vi "Control Panel.vi"(8 "error in (no error)":errorcluster, 11 "TC in":refnum<class "Temperature Controller.lvclass">) -> (0 "error out":errorcluster, 3 "TC out":refnum<class "Temperature Controller.lvclass">)   [LabVIEW 2012, in "Temperature Controller.lvclass"]
uses:
  Temperature Controller.lvclass
  AutoCtl.ctl
  HV Slide Indicator.ctl
  Utility Classes/InstrPtr/InstrPtr.lvclass
  Temperature Controller.lvclass/Temperature Controller.ctl
  Global/Relative Sound Files.vi
  File IO/File IO.lvclass
  Utility Classes/Readable/Readable.lvclass
panel:
  in  "Timer may start":bool
  in  "Fill VTI":bool
  out "log counter":dbl
  in  "Auto":T1
  in  "SET":bool
  in  "New Temp":dbl[unit]=1.3 min=1.3 max=300.0
  in  "Update interval":dbl[unit]=0.5 min=0.1 max=10.0
  out "*itc503":T2
  out "Currently":dbl[unit]
  in  "Stable Sensitivity +-":dbl=0.05 caption="+/-" min=0.0 step=0.1
  out "stable":bool caption="Stable"
  out "Current Set Point":dbl[unit]=6.0 min=0.0 max=305.0
  out "Internal refresh event signal":bool
  in  "Warn At":dbl[unit]
  in  "Comparison":bool
  in  "Alarm?":bool caption="Boolean"
  in  "Time to Fill":dbl[unit]
  out "Time Remaining":string caption="Time"
  in  "Timer?":bool
  out "done?":bool
  in  "clear":bool
  out "Timer start time":timestamp
  in  "Display":dbl[unit]=600.0
  in  "autoscale?":bool=TRUE
  out "Temperature graph":T3(graph)
  out "active":bool
  out "Auto Indicator":T1={"Auto Heater"=FALSE, "Auto Needle"=FALSE, "Auto PID"=TRUE}
  in  "Auto Controls":T4={"Heater"=FALSE, "Needle"=FALSE, "PID"=TRUE}
  out "Ndisbar":T5 caption="Needle Valve              (est. %)" max=100.0 scale=0.0..100.0 scale format="%.1f"
  in  "Ncontrol":dbl(slide) min=0.0 max=100.0 scale=0.0..100.0
  in  "Hcontrol":dbl(slide) min=0.0 max=99.9 scale=0.0..100.0
  out "Hdispbar":T5 caption="Heater" max=100.0 scale=0.0..100.0 scale format="%.1f"
  out "ready?":bool
  in  "endprgm":bool
  # "Temperature Controller"
  # "This will also open the needle valve,\nif that hasn't already been done."
  # "Greater"
  # "Less"
  # "Manual"
  # "Auto"
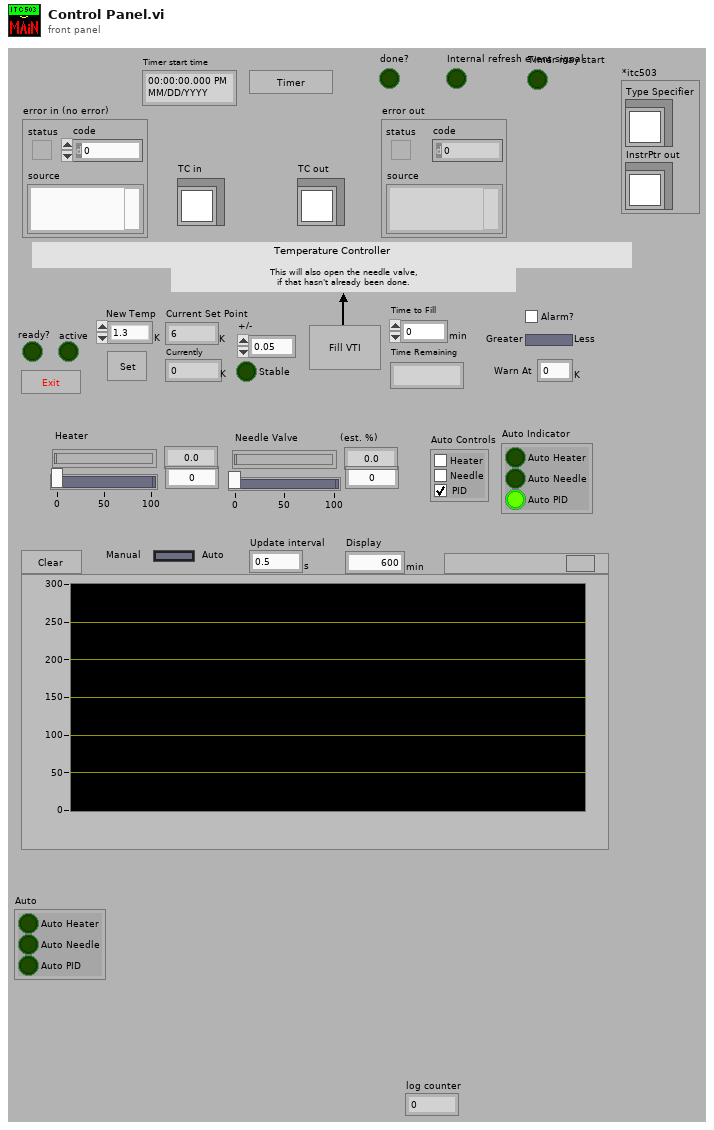
[diagram p1: front panel]
types:
  T1 = typedef "Temperature Controller.lvclass/AutoCtl.ctl" = cluster{"Auto Heater":bool, "Auto Needle":bool, "Auto PID":bool}
  T2 = cluster{"Type Specifier":refnum<class "Temperature Controller.lvclass">, "InstrPtr out":refnum<class "InstrPtr.lvclass">}
  T3 = cluster{"Data Points":cluster{"t":timestamp, "x":dbl}[]}[]
  T4 = cluster{"Heater":bool, "Needle":bool, "PID":bool}
  T5 = typedef "Temperature Controller.lvclass/HV Slide Indicator.ctl" = dbl
  T6 = enum8{"Enabled", "Disabled", "Disabled and Grayed Out"}
  T7 = cluster{"Temperature Controller out":refnum<class "Temperature Controller.lvclass">, "Instrument Pointer":refnum<class "InstrPtr.lvclass">}
  T8 = typedef "ITCIO.ctl" = cluster{"Address":T9, "Version":T10, "Ch 1 dec places":i16, "Ch 2 dec places":i16, "Ch 3 dec places":i16, "Ch1 Name":string, "Ch2 Name":string, "Ch3 Name":string}
  T9 = typedef "OxfordAddress.ctl" = cluster{"Com Port":i32, "ISOBUS Address":i32, "GPIB Address":i16, "Communication":enum16{"RS232", "ISOBUS", "GPIB", "Gateway"}}
  T10 = typedef "ITCVersion.ctl" = enum16{"ITC502", "ITC503", "ITC601"}
  T11 = typedef "Readable.lvclass/TX Graph.ctl" = cluster{"Data Points":cluster{"t":timestamp, "x":dbl}[]}[]
  T12 = cluster{"Data Points":cluster{"t":timestamp, "x":dbl}[]}
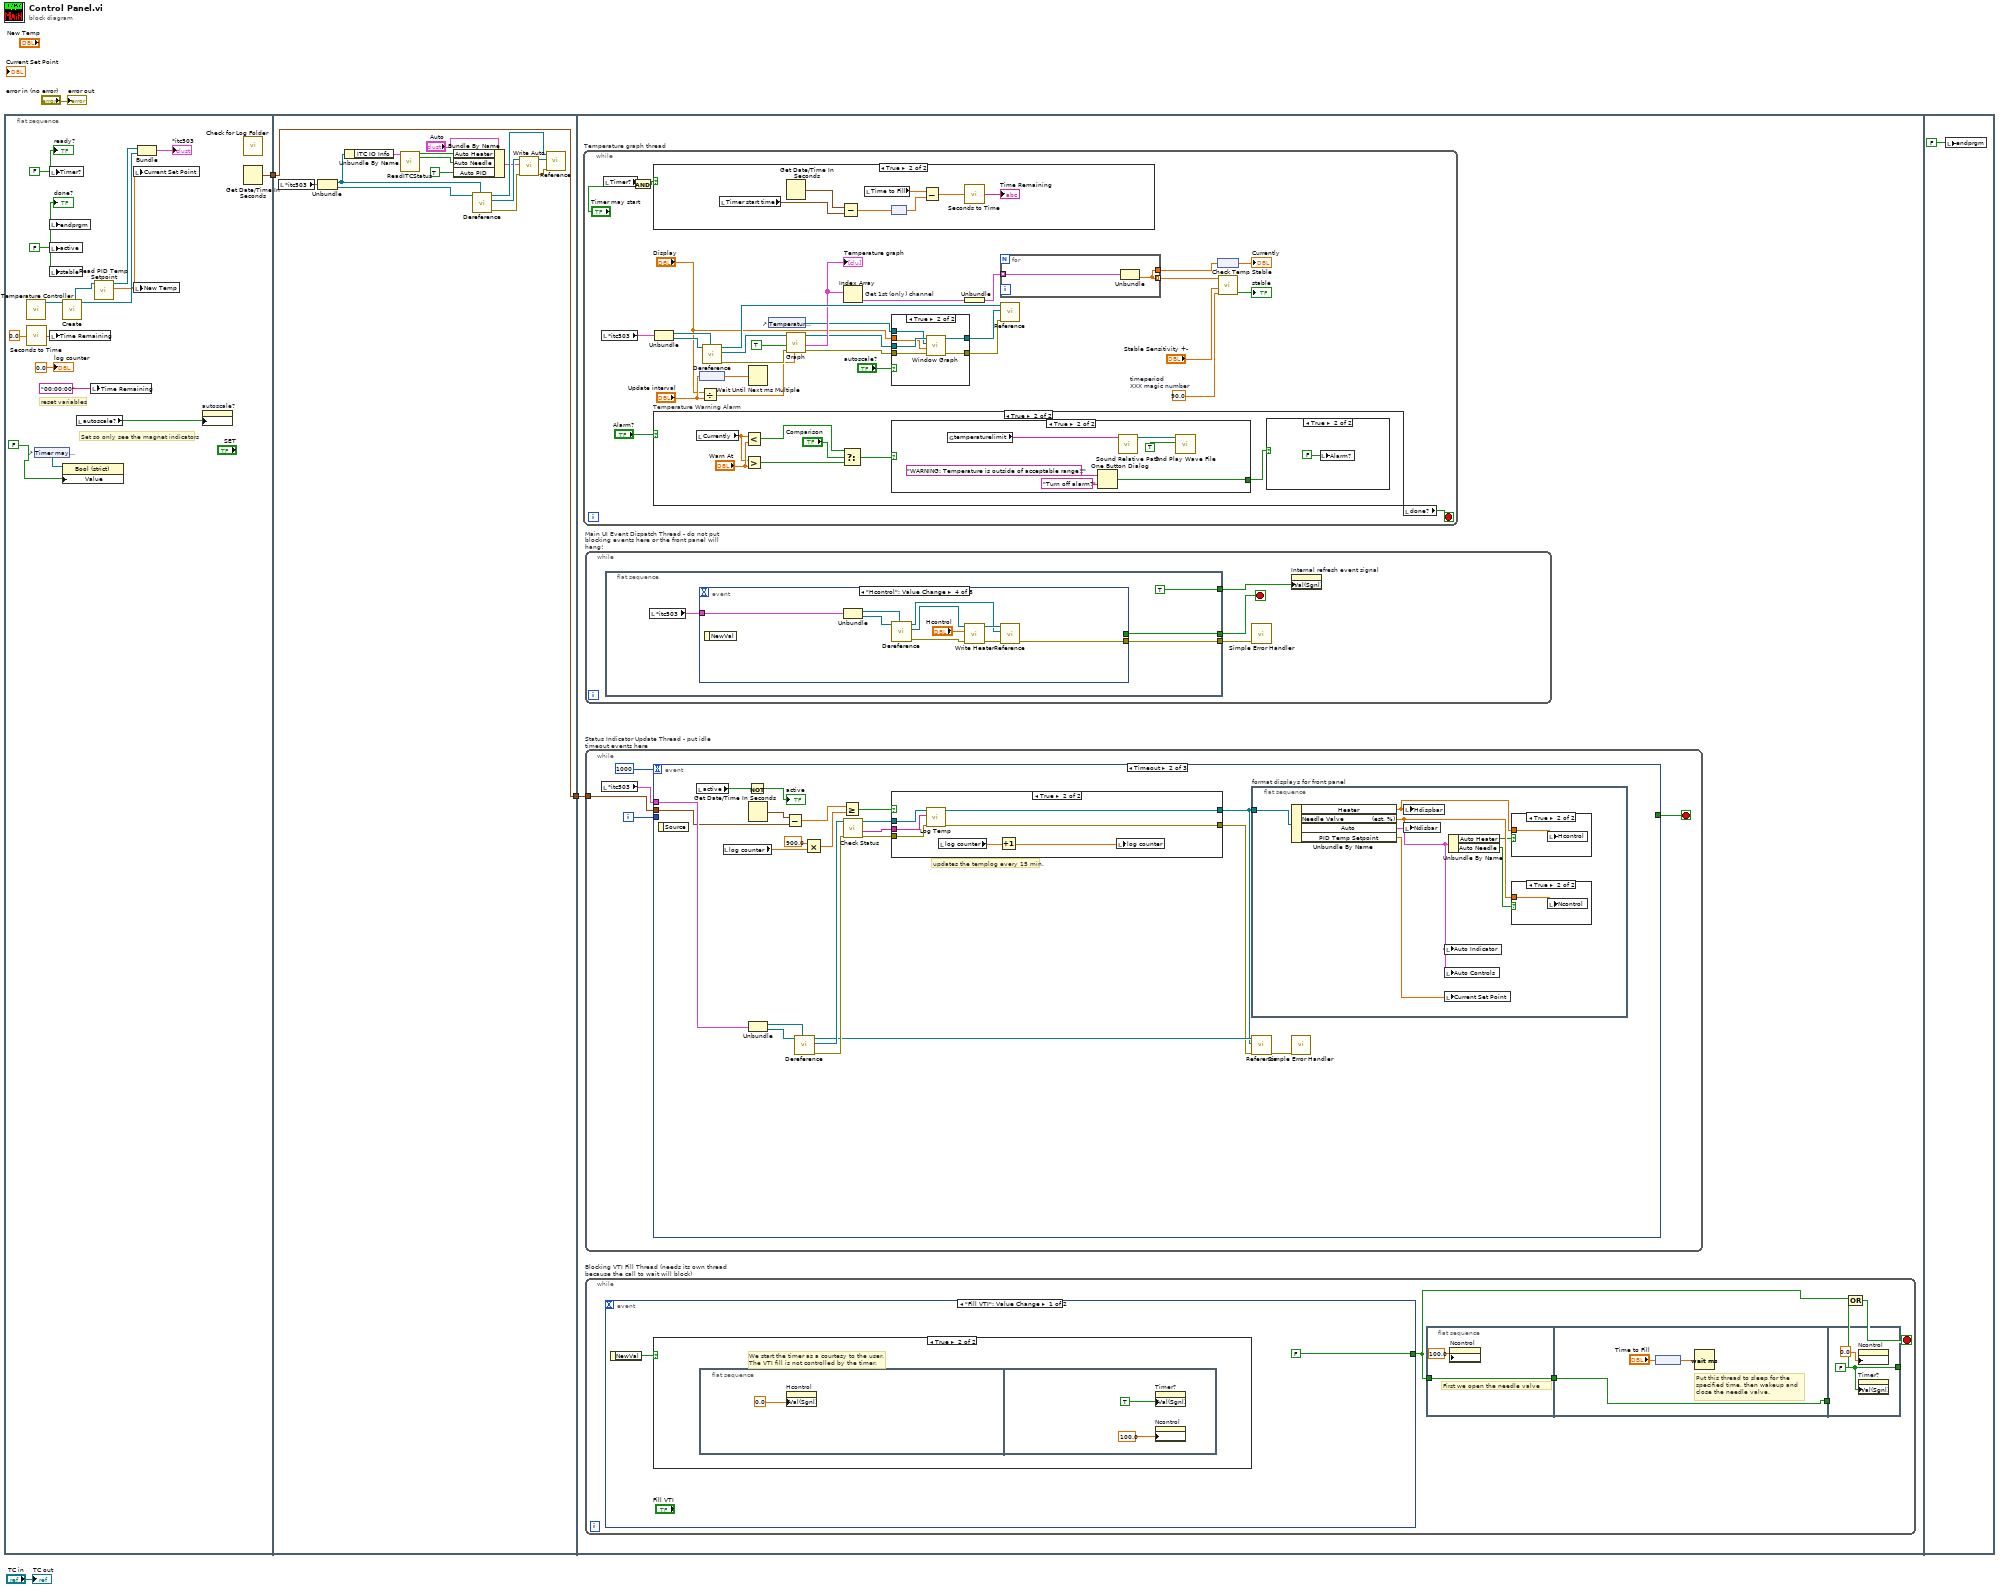
[diagram p0: block diagram]
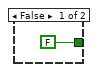
[diagram p6: hidden frame]
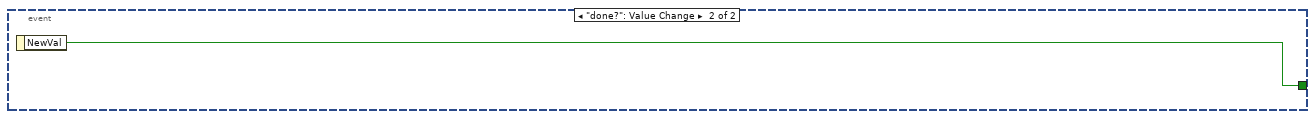
[diagram p8: hidden frame]
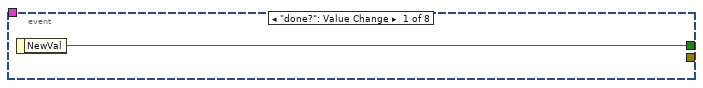
[diagram p9: hidden frame]
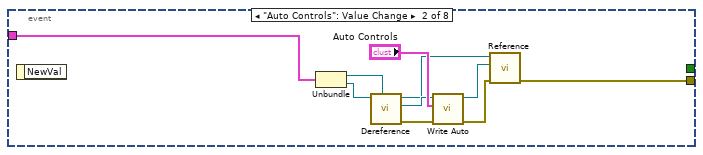
[diagram p10: hidden frame]
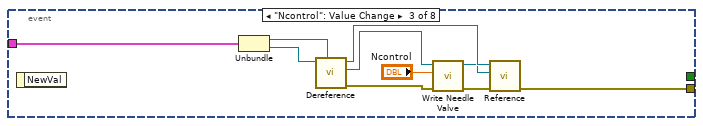
[diagram p11: hidden frame]
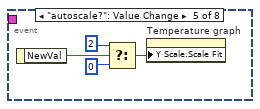
[diagram p12: hidden frame]
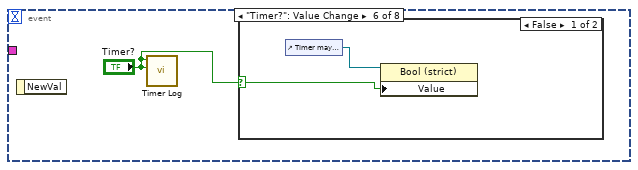
[diagram p13: hidden frame]
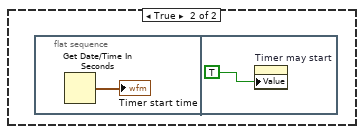
[diagram p14: hidden frame]
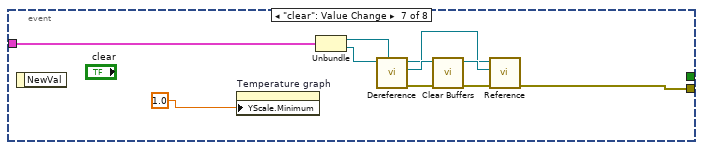
[diagram p15: hidden frame]
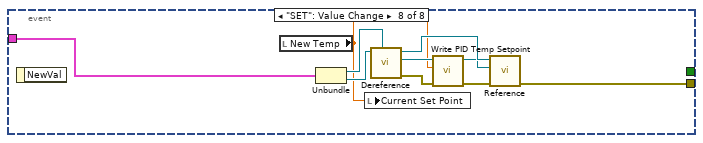
[diagram p16: hidden frame]
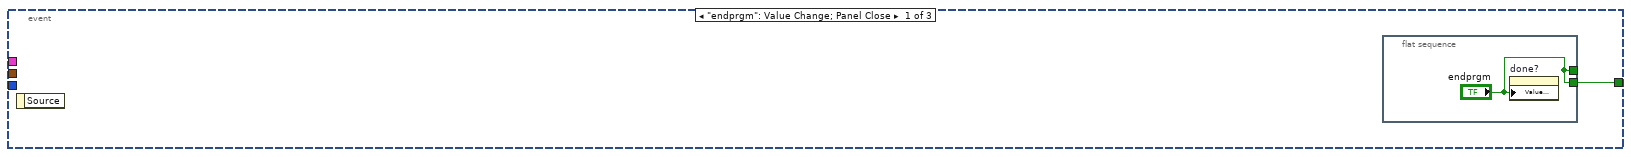
[diagram p17: hidden frame]
diagram:
  n1 = flat-sequence {
    tunnel: [w9] -> w2
    tunnel: w2 -> [w21]
    tunnel: [w21] -> w1
    tunnel: w1 -> [w36]
    frame #0 {
      w20 = FALSE
      w17 = FALSE
      # "Set so only see the magnet indicators"
      # "reset variables"
      n2 = call "Temperature Controller.vi"() -> ("Temperature Controller out"=w16:refnum<class "Temperature Controller.lvclass">)  [unwired: 10 in, 1 out]
      n3 = call "Seconds to Time.vi"("Seconds"=dbl[unit] 0.0) -> ("Time"=w13:string)
      n4 = control-ref of="Timer may start"() -> (w5:refnum<vi>)
      n5 = local write "Timer?"(w20) -> ()
      n6 = local write "endprgm"(w17) -> ()
      n7 = local write "active"(w17) -> ()
      n8 = local write "stable"(w17) -> ()
      n9 = local write "Time Remaining"(w13) -> ()
      n10 = call "Create.vi"("Instrument in"=w16) -> ("Instrument Pointer"=w15:refnum<class "InstrPtr.lvclass">, "Type Specifier"=w11:refnum<class "Temperature Controller.lvclass">)  [unwired: 8 in, 1 out]
      n11 = property on="Property Node" class="Bool (strict)"(reference=w5, "Value"=FALSE) -> ()  [unwired: 1 in, 2 out]
      n12 = local read "autoscale?"() -> (w18:bool)
      n13 = local write "Time Remaining"("00:00:00") -> ()
      n14 = call-dynamic "Read PID Temp Setpoint.vi"("Temperature Controller in"=w11) -> ("PID Temp Setpoint"=w7:dbl[unit], "Temperature Controller out"=w10:refnum<class "Temperature Controller.lvclass">)  [unwired: 8 in, 1 out]
      n15 = local write "Current Set Point"(w7) -> ()
      n16 = local write "New Temp"(w7) -> ()
      n17 = Bundle("Temperature Controller out"=w10, "Instrument Pointer"=w15) -> (→"*itc503":T7)  [unwired: 1 in]
      n18 = property on="autoscale?" class="Bool (strict)"("Value (Signaling)"=w18) -> ()  [unwired: 2 in, 2 out]
      n19 = call "Check for Log Folder.vi"() -> ()  [unwired: 1 out]
      n20 = Get Date/Time In Seconds() -> (seconds since 1Jan1904=w9:timestamp)
      "ready?" <- w20
      "done?" <- w17
      "log counter" <- 0.0 ("log counter")
    }
    frame #1 {
      n21 = local read "*itc503"() -> (w35:T2)
      n22 = Unbundle(w35) -> ("Type Specifier"=w24:refnum<class "Temperature Controller.lvclass">, "InstrPtr out"=w29:refnum<class "InstrPtr.lvclass">)
      n23 = Unbundle By Name(w24) -> ("ITC IO Info"=w23:T8)
      n24 = call "ReadITCStatus.vi"("ITC IO Info"=w23) -> ("Auto heat"=w26:bool, "Auto Needle Valve"=w25:bool)  [unwired: 13 out]
      n25 = Bundle By Name(cluster="Auto", "Auto Heater"=w26, "Auto Needle"=w25, "Auto PID"=TRUE) -> (w27:T1)
      n26 = call "Dereference.vi"("Type Specifier"=w24, "InstrPtr"=w29) -> ("error out"=w34:errorcluster, "Instrument out"=w32:refnum<class "Temperature Controller.lvclass">, "InstrPtr out"=w31:refnum<class "InstrPtr.lvclass">)  [unwired: 7 in]
      n27 = call-dynamic "Write Auto.vi"("error in (no error)"=w34, "Auto"=w27, "Temperature Controller in"=w32) -> ("error out"=w33:errorcluster, "Temperature Controller out"=w30:refnum<class "Temperature Controller.lvclass">)  [unwired: 7 in]
      n28 = call "Reference.vi"("error in (no error)"=w33, "Instrument"=w30, "InstrPtr in"=w31) -> ()  [unwired: 8 in, 1 out]
    }
    frame #2 {
      n29 = while "Temperature graph thread" {
        stop <- w48 stop-if-true
        w60 = 90.0  # timeperiod XXX magic number
        n30 = local read "*itc503"() -> (w56:T2)
        n31 = local read "Timer?"() -> (w49:bool)
        n32 = And(x=w49, y="Timer may start") -> (x .and. y?=w38:bool)
        n33 = case shown="True" w38 {
          frame False {
          }
          frame True {
            n34 = local read "Timer start time"() -> (w73:timestamp)
            n35 = Get Date/Time In Seconds ("jkl;jkljkl")() -> (seconds since 1Jan1904=w74:timestamp)
            n36 = Subtract(x=w74, y=w73) -> (x-y=w76:dbl)
            n37 = local read "Time to Fill"() -> (w70:dbl[unit])
            n38 = node(w76) -> (w72:dbl[unit])
            n39 = Subtract(x=w70, y=w72) -> (x-y=w71:dbl[unit])
            n40 = call "Seconds to Time.vi"("Seconds"=w71) -> ("Time"=→"Time Remaining":string)
          }
        }
        n41 = case "Temperature Warning Alarm" shown="True" "Alarm?" {
          frame False {
          }
          frame True {
            n42 = local read "Currently"() -> (w86:dbl[unit])
            n43 = Less?(x=w86, y="Warn At") -> (x < y?=w90:bool)
            n44 = Greater?(x=w86, y="Warn At") -> (0:w89:bool)
            n45 = Select(t=w90, s="Comparison", f=w89) -> (s? t:f=w88:bool)
            n46 = case shown="True" w88 {
              tunnel: [FALSE ("true") w95] -> w85
              frame False {
              }
              frame True {
                n47 = global read "Relative Sound Files.vi" "temperaturelimit"() -> (w98:string)
                n48 = One Button Dialog(message="WARNING: Temperature is outside of acceptable range!!", button name ("OK")="Turn off alarm?") -> (true=w95:bool)
                n49 = call "Sound Relative Path.vi"("Sound"=w98) -> ("Relative Path"=w97:path)  [unwired: 10 in]
                n50 = call <vilib>:"Snd Play Wave File.vi"("wait until finish (T)"=TRUE, "wave file path"=w97) -> ()  [unwired: 1 in, 9 out]
              }
            }
            n51 = case shown="True" w85 {
              frame False {
              }
              frame True {
                n52 = local write "Alarm?"(FALSE ("Alarm?")) -> ()
              }
            }
          }
        }
        n53 = Unbundle(w56) -> ("Type Specifier"=w61:refnum<class "Temperature Controller.lvclass">, "InstrPtr out"=w62:refnum<class "InstrPtr.lvclass">)
        n54 = node("Update interval") -> (w47:dbl)
        n55 = Divide(x="Display", y="Update interval") -> (x/y=w45:dbl)
        n56 = call "Dereference.vi"("Type Specifier"=w61, "InstrPtr"=w62) -> ("error out"=w65:errorcluster, "Instrument out"=w64:refnum<class "Temperature Controller.lvclass">, "InstrPtr out"=w63:refnum<class "InstrPtr.lvclass">)  [unwired: 7 in]
        n57 = Wait Until Next ms Multiple(millisecond multiple=w47) -> ()  [unwired: 1 out]
        n58 = control-ref of="Temperature graph"() -> (w40:refnum<vi>)
        n59 = call-dynamic "Graph.vi"("Ring size (points) (1024)"=w45, "error in (no error)"=w65, "Store Ring? (f)"=TRUE, "Readable in"=w64) -> ("error out"=w44:errorcluster, "Ring Buffers"=w55:T11, "Readable out"=w43:refnum<class "Temperature Controller.lvclass">)  [unwired: 1 in, 4 out]
        "Temperature graph" <- w55
        n60 = Index Array "Get 1st (only) channel"(array=w55) -> (element=w54:T12)  [unwired: 1 in]
        n61 = case shown="True" "autoscale?" {
          tunnel: w44 -> [w77 w84]
          tunnel: w43 -> [w78 w83]
          tunnel: [w78 w82] -> w42
          tunnel: [w77 w81] -> w41
          tunnel: w40 -> [_ w80]
          tunnel: "Display" -> [_ w79]
          frame False {
          }
          frame True {
            n62 = call-dynamic "Window Graph.vi"("error in (no error)"=w84, "Window"=w79, "Graph ref"=w80, "Readable in"=w83) -> ("error out"=w81:errorcluster, "Readable out"=w82:refnum<class "Temperature Controller.lvclass">)  [unwired: 6 in]
          }
        }
        n63 = Unbundle(w54) -> ("Data Points"=w53:cluster{"t":timestamp, "x":dbl}[])
        n64 = for {
          tunnel: w53 -> [w69] mode=indexing
          tunnel: [w68] -> w52 mode=indexing
          tunnel: [w68] -> w51
          n65 = Unbundle(w69) -> ("x"=w68:dbl)  [unwired: 1 out]
        }
        n66 = call "Reference.vi"("error in (no error)"=w41, "Instrument"=w42, "InstrPtr in"=w63) -> ()  [unwired: 8 in, 1 out]
        n67 = node(w51) -> (→"Currently":dbl[unit])
        n68 = call "Check Temp Stable.vi"("timeperiod"=w60, "sens"="Stable Sensitivity +-", "temparray"=w52) -> ("stable"=→"stable":bool)  [unwired: 8 in]
        n69 = local read "done?"() -> (w48:bool)
      }
      n70 = while "Main UI Event Dispatch Thread - do not put blocking events here or the front panel will hang!" {
        stop <- w120 stop-if-true
        n71 = flat-sequence {
          tunnel: [w124] -> w119
          tunnel: [w123] -> w120
          tunnel: [TRUE ("Value (Signaling)")] -> w118
          frame #0 {
            n72 = local read "*itc503"() -> (w122:T2)
            n73 = event shown="[3] \"Hcontrol\": Value Change" {
              selector: _ -> [_ _ _ _ _ _ _ _]
              dyn-events: _ -> [_ _ _ _ _ _ _ _]
              timeout: _ -> [_ _ _ _ _ _ _ _]
              tunnel: [w125 _ _ _ _ _ _ _] -> w123
              tunnel: w122 -> [_ w131 w142 w151 _ _ w169 w181]
              tunnel: [_ w132 w143 w152 _ _ w166 w182] -> w124
              event "done?": Value Change {
                n74 = event-data() -> ("NewVal"=w125:bool)  [unwired: 1 out]
              }
              event "Auto Controls": Value Change {
                n75 = event-data() -> ()  [unwired: 2 out]
                n76 = Unbundle(w131) -> ("Type Specifier"=w127:refnum<class "Temperature Controller.lvclass">, "InstrPtr out"=w126:refnum<class "InstrPtr.lvclass">)
                n77 = call "Dereference.vi"("Type Specifier"=w127, "InstrPtr"=w126) -> ("error out"=w134:errorcluster, "Instrument out"=w130:refnum<class "Temperature Controller.lvclass">, "InstrPtr out"=w129:refnum<class "InstrPtr.lvclass">)  [unwired: 7 in]
                n78 = call-dynamic "Write Auto.vi"("error in (no error)"=w134, "Auto"="Auto Controls", "Temperature Controller in"=w130) -> ("error out"=w133:errorcluster, "Temperature Controller out"=w128:refnum<class "Temperature Controller.lvclass">)  [unwired: 7 in]
                n79 = call "Reference.vi"("error in (no error)"=w133, "Instrument"=w128, "InstrPtr in"=w129) -> ("error out"=w132:errorcluster)  [unwired: 8 in]
              }
              event "Ncontrol": Value Change {
                n80 = event-data() -> ()  [unwired: 2 out]
                n81 = Unbundle(w142) -> ("Type Specifier"=w138:refnum<class "Temperature Controller.lvclass">, "InstrPtr out"=w137:refnum<class "InstrPtr.lvclass">)
                n82 = call "Dereference.vi"("Type Specifier"=w138, "InstrPtr"=w137) -> ("error out"=w144:errorcluster, "Instrument out"=w141:refnum<class "Temperature Controller.lvclass">, "InstrPtr out"=w140:refnum<class "InstrPtr.lvclass">)  [unwired: 7 in]
                n83 = call-dynamic "Write Needle Valve.vi"("error in (no error)"=w144, "Heater"="Ncontrol", "Temperature Controller in"=w141) -> ("error out"=w145:errorcluster, "Temperature Controller out"=w139:refnum<class "Temperature Controller.lvclass">)  [unwired: 7 in]
                n84 = call "Reference.vi"("error in (no error)"=w145, "Instrument"=w139, "InstrPtr in"=w140) -> ("error out"=w143:errorcluster)  [unwired: 8 in]
              }
              event "Hcontrol": Value Change {
                n85 = event-data() -> ()  [unwired: 2 out]
                n86 = Unbundle(w151) -> ("Type Specifier"=w146:refnum<class "Temperature Controller.lvclass">, "InstrPtr out"=w147:refnum<class "InstrPtr.lvclass">)
                n87 = call "Dereference.vi"("Type Specifier"=w146, "InstrPtr"=w147) -> ("error out"=w154:errorcluster, "Instrument out"=w150:refnum<class "Temperature Controller.lvclass">, "InstrPtr out"=w149:refnum<class "InstrPtr.lvclass">)  [unwired: 7 in]
                n88 = call-dynamic "Write Heater.vi"("error in (no error)"=w154, "Heater"="Hcontrol", "Temperature Controller in"=w150) -> ("error out"=w153:errorcluster, "Temperature Controller out"=w148:refnum<class "Temperature Controller.lvclass">)  [unwired: 7 in]
                n89 = call "Reference.vi"("error in (no error)"=w153, "Instrument"=w148, "InstrPtr in"=w149) -> ("error out"=w152:errorcluster)  [unwired: 8 in]
              }
              event "autoscale?": Value Change {
                n90 = event-data() -> ("NewVal"=w156:bool)  [unwired: 1 out]
                n91 = Select(t=2, s=w156, f=0) -> (s? t:f=w159:i32)
                n92 = property on="Temperature graph" class="XYGraph (strict)"("Y Scale.Scale Fit"=w159) -> ()  [unwired: 2 in, 2 out]
              }
              event "Timer?": Value Change {
                n93 = event-data() -> ()  [unwired: 2 out]
                n94 = call "Timer Log.vi"("flag"="Timer?", "toggle"="Timer?") -> ()  [unwired: 10 out]
                n95 = case shown="False" "Timer?" {
                  selector: "Timer?" -> [w162 _]
                  frame False {
                    n96 = control-ref of="Timer may start"() -> (w161:refnum<vi>)
                    n97 = property on="Property Node" class="Bool (strict)"(reference=w161, "Value"=w162) -> ()  [unwired: 1 in, 2 out]
                  }
                  frame True {
                    n98 = flat-sequence {
                      frame #0 {
                        n99 = Get Date/Time In Seconds() -> (seconds since 1Jan1904=→"Timer start time":timestamp)
                      }
                      frame #1 {
                        n100 = property on="Timer may start" class="Bool (strict)"("Value"=TRUE ("Value (Signaling)")) -> ()  [unwired: 2 in, 2 out]
                      }
                    }
                  }
                }
              }
              event "clear": Value Change {
                n101 = event-data() -> ()  [unwired: 2 out]
                n102 = property on="Temperature graph" class="XYGraph (strict)"("YScale.Minimum"=1.0) -> ()  [unwired: 2 in, 2 out]
                n103 = Unbundle(w169) -> ("Type Specifier"=w170:refnum<class "Temperature Controller.lvclass">, "InstrPtr out"=w171:refnum<class "InstrPtr.lvclass">)
                n104 = call "Dereference.vi"("Type Specifier"=w170, "InstrPtr"=w171) -> ("error out"=w168:errorcluster, "Instrument out"=w174:refnum<class "Temperature Controller.lvclass">, "InstrPtr out"=w172:refnum<class "InstrPtr.lvclass">)  [unwired: 7 in]
                n105 = call "Clear Buffers.vi"("error in (no error)"=w168, "Readable in"=w174) -> ("error out"=w167:errorcluster, "Readable out"=w173:refnum<class "Temperature Controller.lvclass">)  [unwired: 8 in]
                n106 = call "Reference.vi"("error in (no error)"=w167, "Instrument"=w173, "InstrPtr in"=w172) -> ("error out"=w166:errorcluster)  [unwired: 8 in]
              }
              event "SET": Value Change {
                n107 = event-data() -> ()  [unwired: 2 out]
                n108 = local read "New Temp"() -> (w175:dbl[unit])
                n109 = Unbundle(w181) -> ("Type Specifier"=w177:refnum<class "Temperature Controller.lvclass">, "InstrPtr out"=w176:refnum<class "InstrPtr.lvclass">)
                n110 = local write "Current Set Point"(w175) -> ()
                n111 = call "Dereference.vi"("Type Specifier"=w177, "InstrPtr"=w176) -> ("error out"=w183:errorcluster, "Instrument out"=w179:refnum<class "Temperature Controller.lvclass">, "InstrPtr out"=w180:refnum<class "InstrPtr.lvclass">)  [unwired: 7 in]
                n112 = call-dynamic "Write PID Temp Setpoint.vi"("error in (no error)"=w183, "PID Temp Setpoint"=w175, "Temperature Controller in"=w179) -> ("error out"=w184:errorcluster, "Temperature Controller out"=w178:refnum<class "Temperature Controller.lvclass">)  [unwired: 7 in]
                n113 = call "Reference.vi"("error in (no error)"=w184, "Instrument"=w178, "InstrPtr in"=w180) -> ("error out"=w182:errorcluster)  [unwired: 8 in]
              }
            }
          }
        }
        n114 = call <vilib>:"Simple Error Handler.vi"("error in (no error)"=w119) -> ()  [unwired: 4 in, 5 out]
        n115 = property on="Internal refresh event signal" class="Bool (strict)"("Val(Sgnl)"=w118) -> ()  [unwired: 2 in, 2 out]
      }
      n116 = while "Status Indicator Update Thread - put idle timeout events here" {
        tunnel: w36 -> [w185]
        i -> [w187]
        stop <- w188 stop-if-true
        n117 = local read "*itc503"() -> (w186:T2)
        n118 = event shown="[1] Timeout" {
          selector: _ -> [_ _ _]
          dyn-events: _ -> [_ _ _]
          timeout: 1000 -> [_ _ _]
          tunnel: [w190 _ _] -> w188
          tunnel: w187 -> [_ _ _]
          tunnel: w186 -> [_ w210 w239]
          tunnel: w185 -> [_ w196 _]
          event "endprgm": Value Change; Panel Close {
            n119 = event-data() -> ()  [unwired: 2 out]
            n120 = flat-sequence {
              tunnel: ["endprgm"] -> _
              tunnel: ["endprgm"] -> w190
              frame #0 {
                n121 = property on="done?" class="Bool (strict)"("Value (Signaling)"="endprgm") -> ()  [unwired: 2 in, 2 out]
              }
            }
          }
          event Timeout {
            # "updates the templog every 15 min."
            n122 = event-data() -> ()  [unwired: 2 out]
            n123 = local read "active"() -> (w212:bool)
            n124 = local read "log counter"() -> (w194:dbl)
            n125 = Not(x=w212) -> (.not. x?=→"active":bool)
            n126 = Get Date/Time In Seconds() -> (seconds since 1Jan1904=w197:timestamp)
            n127 = Unbundle(w210) -> ("Type Specifier"=w206:refnum<class "Temperature Controller.lvclass">, "InstrPtr out"=w207:refnum<class "InstrPtr.lvclass">)
            n128 = Subtract(x=w197, y=w196) -> (x-y=w192:dbl)
            n129 = call "Dereference.vi"("Type Specifier"=w206, "InstrPtr"=w207) -> ("error out"=w209:errorcluster, "Instrument out"=w208:refnum<class "Temperature Controller.lvclass">, "InstrPtr out"=w205:refnum<class "InstrPtr.lvclass">)  [unwired: 7 in]
            n130 = Multiply(x=900.0 ("y"), y=w194) -> (x*y=w193:dbl)
            n131 = Greater Or Equal?(x=w192, y=w193) -> (x >= y?=w199:bool)
            n132 = call-dynamic "Check Status.vi"("error in (no error)"=w209, "Temperature Controller in"=w208) -> ("error out"=w202:errorcluster, "Status"=w198:string, "Temperature Controller out"=w204:refnum<class "Temperature Controller.lvclass">)  [unwired: 6 in, 1 out]
            n133 = case shown="True" w199 {
              tunnel: w204 -> [w214 w221]
              tunnel: [w214 w220] -> w203
              tunnel: w202 -> [w213 w219]
              tunnel: [w213 w218] -> w201
              tunnel: w198 -> [_ w217]
              frame False {
              }
              frame True {
                n134 = call-dynamic "Log Temp.vi"("error in (no error)"=w219, "Status string"=w217, "Temperature Controller in"=w221) -> ("error out"=w218:errorcluster, "Temperature Controller out"=w220:refnum<class "Temperature Controller.lvclass">)  [unwired: 7 in]
                n135 = local read "log counter"() -> (w216:dbl)
                n136 = Increment(x=w216) -> (x+1=w215:dbl)
                n137 = local write "log counter"(w215) -> ()
              }
            }
            n138 = flat-sequence "format displays for front panel" {
              tunnel: w203 -> [w228]
              frame #0 {
                n139 = Unbundle By Name(w228) -> ("Heater"=w226:T5, "Needle Valve              (est. %)"=w225:T5, "Auto"=w224:T1, "PID Temp Setpoint"=w227:dbl[unit])
                n140 = local write "Hdispbar"(w226) -> ()
                n141 = local write "Ndisbar"(w225) -> ()
                n142 = local write "Auto Indicator"(w224) -> ()
                n143 = local write "Auto Controls"(w224) -> ()
                n144 = local write "Current Set Point"(w227) -> ()
                n145 = Unbundle By Name(w224) -> ("Auto Heater"=w223:bool, "Auto Needle"=w222:bool)
                n146 = case shown="True" w223 {
                  tunnel: w226 -> [_ w230]
                  frame False {
                  }
                  frame True {
                    n147 = local write "Hcontrol"(w230) -> ()
                  }
                }
                n148 = case shown="True" w222 {
                  tunnel: w225 -> [_ w229]
                  frame False {
                  }
                  frame True {
                    n149 = local write "Ncontrol"(w229) -> ()
                  }
                }
              }
            }
            n150 = call "Reference.vi"("error in (no error)"=w201, "Instrument"=w203, "InstrPtr in"=w205) -> ("error out"=w200:errorcluster)  [unwired: 8 in]
            n151 = call <vilib>:"Simple Error Handler.vi"("error in (no error)"=w200) -> ()  [unwired: 4 in, 5 out]
          }
          event "Internal refresh event signal": Value Change {
            # "min = max - window\nmax = now"
            # "read indicators"
            # "check whats on and read settings"
            n152 = event-data() -> ()  [unwired: 2 out]
            n153 = Unbundle(w239) -> ("Type Specifier"=w237:refnum<class "Temperature Controller.lvclass">, "InstrPtr out"=w236:refnum<class "InstrPtr.lvclass">)
            n154 = call "Dereference.vi"("Type Specifier"=w237, "InstrPtr"=w236) -> ("error out"=w233:errorcluster, "Instrument out"=w235:refnum<class "Temperature Controller.lvclass">, "InstrPtr out"=w234:refnum<class "InstrPtr.lvclass">)  [unwired: 7 in]
            n155 = call-dynamic "Check Status.vi"("error in (no error)"=w233, "Temperature Controller in"=w235) -> ("error out"=w232:errorcluster, "Ready?"=w238:bool, "Temperature Controller out"=w231:refnum<class "Temperature Controller.lvclass">)  [unwired: 6 in, 1 out]
            n156 = local write "ready?"(w238) -> ()
            n157 = call "Reference.vi"("error in (no error)"=w232, "Instrument"=w231, "InstrPtr in"=w234) -> ()  [unwired: 8 in, 1 out]
            n158 = flat-sequence "format displays for front panel" {
              tunnel: w231 -> [w245]
              frame #0 {
                n159 = Unbundle By Name(w245) -> ("Heater"=w249:T5, "Needle Valve              (est. %)"=w246:T5, "Auto"=w248:T1, "PID Temp Setpoint"=w244:dbl[unit])
                "Auto Indicator" <- w248
                "Ndisbar" <- w246
                "Hdispbar" <- w249
                n160 = local write "Auto Controls"(w248) -> ()
                n161 = local write "Current Set Point"(w244) -> ()
                n162 = Unbundle By Name(w248) -> ("Auto Heater"=w250:bool)
                n163 = Unbundle By Name(w248) -> ("Auto Needle"=w247:bool)
                n164 = case shown="True" w250 {
                  tunnel: w249 -> [_ w252]
                  frame False {
                  }
                  frame True {
                    n165 = local write "Hcontrol"(w252) -> ()
                  }
                }
                n166 = case shown="True" w247 {
                  tunnel: w246 -> [_ w251]
                  frame False {
                  }
                  frame True {
                    n167 = local write "Ncontrol"(w251) -> ()
                  }
                }
              }
            }
            n168 = flat-sequence "Disable controls if unit is powered off" {
              tunnel: w238 -> [w242]
              frame #0 {
                n169 = Select(t=T6."Enabled" ("Disabled"), s=w242, f=T6."Disabled and Grayed Out" ("Disabled")) -> (s? t:f=w243:T6)
                n170 = property on="Current Set Point" class="DigNum (strict)"("Disabled"=w243) -> ()  [unwired: 2 in, 2 out]
                n171 = property on="Hdispbar" class="Slide (strict)"("Disabled"=w243) -> ()  [unwired: 2 in, 2 out]
                n172 = property on="Hcontrol" class="Slide (strict)"("Disabled"=w243) -> ()  [unwired: 2 in, 2 out]
                n173 = property on="Ncontrol" class="Slide (strict)"("Disabled"=w243) -> ()  [unwired: 2 in, 2 out]
                n174 = property on="Ndisbar" class="Slide (strict)"("Disabled"=w243) -> ()  [unwired: 2 in, 2 out]
                n175 = property on="Stable Sensitivity +-" class="DigNum (strict)"("Disabled"=w243) -> ()  [unwired: 2 in, 2 out]
                n176 = property on="Auto Controls" class="Clust (strict)"("Disabled"=w243) -> ()  [unwired: 2 in, 2 out]
                n177 = property on="Auto Indicator" class="Clust (strict)"("Disabled"=w243) -> ()  [unwired: 2 in, 2 out]
                n178 = property on="stable" class="Bool (strict)"("Disabled"=w243) -> ()  [unwired: 2 in, 2 out]
              }
            }
          }
        }
      }
      n179 = while "Blocking VTI Fill Thread (needs its own thread because the call to wait will block)" {
        stop <- w103 stop-if-true
        n180 = event shown="[0] \"Fill VTI\": Value Change" {
          selector: _ -> [_ _]
          dyn-events: _ -> [_ _]
          timeout: _ -> [_ _]
          tunnel: [FALSE ("NewVal") w117] -> w101
          event "Fill VTI": Value Change {
            n181 = event-data() -> ("NewVal"=w112:bool)  [unwired: 1 out]
            n182 = case shown="True" w112 {
              frame False {
              }
              frame True {
                # "We start the timer as a courtesy to the user.\nThe VTI fill is not controlled by the timer."
                n183 = flat-sequence {
                  frame #0 {
                    n184 = property on="Hcontrol" class="Slide (strict)"("Val(Sgnl)"=0.0 ("Ncontrol")) -> ()  [unwired: 2 in, 2 out]
                  }
                  frame #1 {
                    n185 = property on="Timer?" class="Bool (strict)"("Val(Sgnl)"=TRUE ("Value (Signaling)")) -> ()  [unwired: 2 in, 2 out]
                    n186 = property on="Ncontrol" class="Slide (strict)"("Value (Signaling)"=100.0 ("Ncontrol")) -> ()  [unwired: 2 in, 2 out]
                  }
                }
              }
            }
          }
          event "done?": Value Change {
            n187 = event-data() -> ("NewVal"=w117:bool)  [unwired: 1 out]
          }
        }
        n188 = flat-sequence {
          tunnel: w101 -> [w106]
          tunnel: [w106] -> w100
          tunnel: [w107] -> w104
          tunnel: w100 -> [w107]
          tunnel: w104 -> [_]
          tunnel: [w110] -> w102
          frame #0 {
            # "First we open the needle valve"
            n189 = property on="Ncontrol" class="Slide (strict)"("Value (Signaling)"=100.0 ("Ncontrol")) -> ()  [unwired: 2 in, 2 out]
          }
          frame #1 {
            # "Put this thread to sleep for the specified time, then wakeup and close the needle valve."
            n190 = node("Time to Fill") -> (w108:dbl)
            n191 = Wait (ms)(milliseconds to wait=w108) -> ()  [unwired: 1 out]
          }
          frame #2 {
            w110 = FALSE ("Value (Signaling)")
            n192 = property on="Ncontrol" class="Slide (strict)"("Value (Signaling)"=0.0 ("Ncontrol")) -> ()  [unwired: 2 in, 2 out]
            n193 = property on="Timer?" class="Bool (strict)"("Val(Sgnl)"=w110) -> ()  [unwired: 2 in, 2 out]
          }
        }
        n194 = Or(x=w101, y=w102) -> (x .or. y?=w103:bool)
      }
    }
    frame #3 {
      n195 = local write "endprgm"(FALSE) -> ()
    }
  }
  "error out" <- "error in (no error)"
  "TC out" <- "TC in"
